vi "5.vi"(2 "Boolean":bool, 11 "Numeric":dbl) -> (3 "String":string)   [LabVIEW 2023]
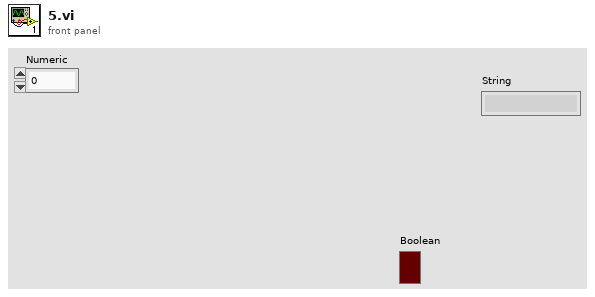
[diagram p1: front panel]
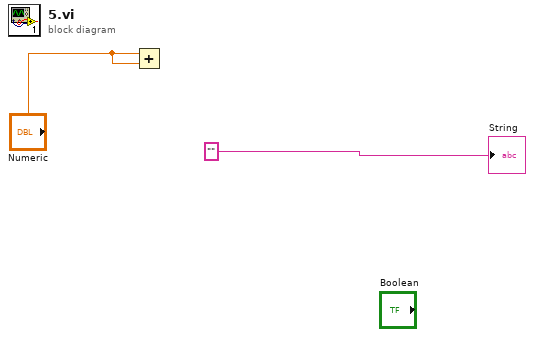
[diagram p0: block diagram]
diagram:
  n1 = Add(x="Numeric", y="Numeric") -> ()  [unwired: 1 out]
  "String" <- "" ("String")
